vi "GET_CAPTURE.vi"(3 "Option Edge":dbl=1.0 min=1.0 max=3.0, 4 "error in (no error)":errorcluster, 5 "VISA resource name":refnum<visa-resource-name>) -> (0 "error out":errorcluster, 1 "(hi.lo) Period":i16, 2 "VISA resource Salida":refnum<visa-resource-name>)   [LabVIEW 2011]
panel:
  out "unsigned byte array":u8[](array[numeric])
  out "return count":u32
  out "Read get_Capture command":u8[](array[numeric])
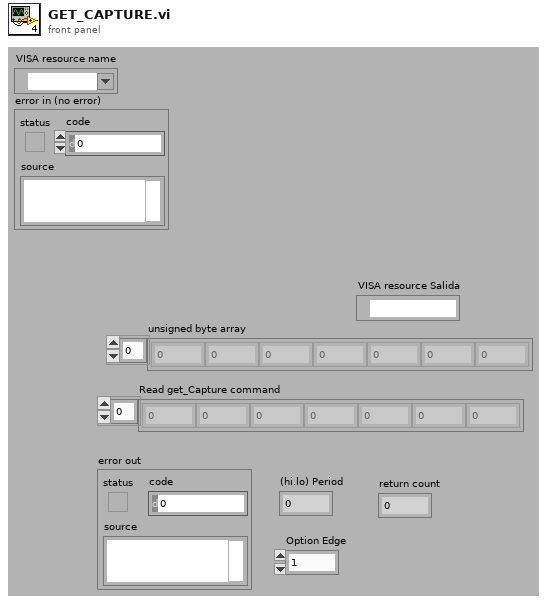
[diagram p1: front panel]
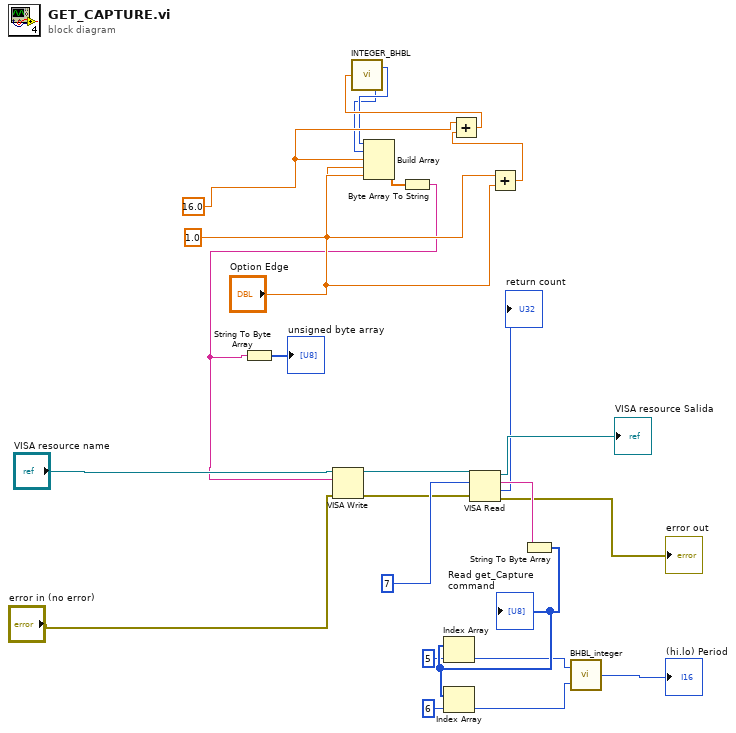
[diagram p0: block diagram]
diagram:
  w8 = 1.0 ("element")
  w6 = 16.0 ("element")
  n1 = Add(x=w8, y="Option Edge") -> (x+y=w7:dbl)
  n2 = Add(x=w6, y=w7) -> (x+y=w5:dbl)
  n3 = call "INTEGER_BHBL.vi"("int16"=w5) -> ("Lvalue"=w3:u8, "HValue"=w4:u8)
  n4 = Build Array(w4, w3, w6, w8, "Option Edge") -> (w19:dbl[])
  n5 = Byte Array To String(unsigned byte array=w19) -> (string=w2:string)
  n6 = String To Byte Array(string=w2) -> (unsigned byte array=→"unsigned byte array":u8[])
  n7 = VISA Write(VISA resource name="VISA resource name", write buffer=w2, error in (no error)="error in (no error)") -> (VISA resource name out=w20:refnum<visa-resource-name>, error out=w22:errorcluster)  [unwired: 1 out]
  n8 = VISA Read(VISA resource name=w20, byte count=u32 7, error in (no error)=w22) -> (VISA resource name out=→"VISA resource Salida":refnum<visa-resource-name>, read buffer=w24:string, return count=→"return count":u32, error out=→"error out":errorcluster)
  n9 = String To Byte Array(string=w24) -> (unsigned byte array=w17:u8[])
  "Read get_Capture command" <- w17
  n10 = Index Array(array=w17, index=5) -> (element=w14:u8)
  n11 = Index Array(array=w17, index=6) -> (element=w13:u8)
  n12 = call "BHBL_integer.vi"("lo(x)"=w13, "hi(x)"=w14) -> ("(hi.lo)"=→"(hi.lo) Period":i16)
